vi "Loop (DMA) BAD CHANNELS.vi"(8 "Error IN":errorcluster, 9 "Stop":refnum<vi>, 10 "Sample Rate":u32, 11 "FPGA Ref":T1) -> (0 "Error OUT":errorcluster, 3 "FPGA Ref OUT":T1)   [LabVIEW 2019]
uses:
  <vilib>/rvi/interface/nirviMethod/nirviMethod.xnode
  <vilib>/rvi/errors/niLvFpgaMergeErrorWithErrorCode.vi
  Real-Time/Controls/RT FIFO Mode.ctl
  Type Defs/Pump Data Mode.ctl
  Controls/FPGA_Reference.ctl
  <vilib>/FPGAPlugInAG/Dynamic/niLvFpga_ReadFifo_Dynamic.vi
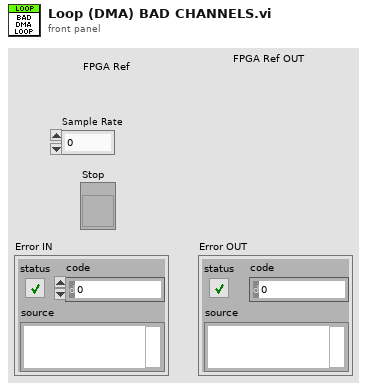
[diagram p1: front panel]
types:
  T1 = typedef "FPGA_Reference.ctl" = refnum<k20>
  T2 = typedef "Pump Data Mode.ctl" = enum16{"Read", "Write Data", "Write Cal", "Write Watlow Data", "Write Pressure Offsets", "Write Initial Times", "Write Pumps Present"}
  T3 = typedef "RT FIFO Mode.ctl" = enum16{"Create", "Write", "Read", "Delete"}
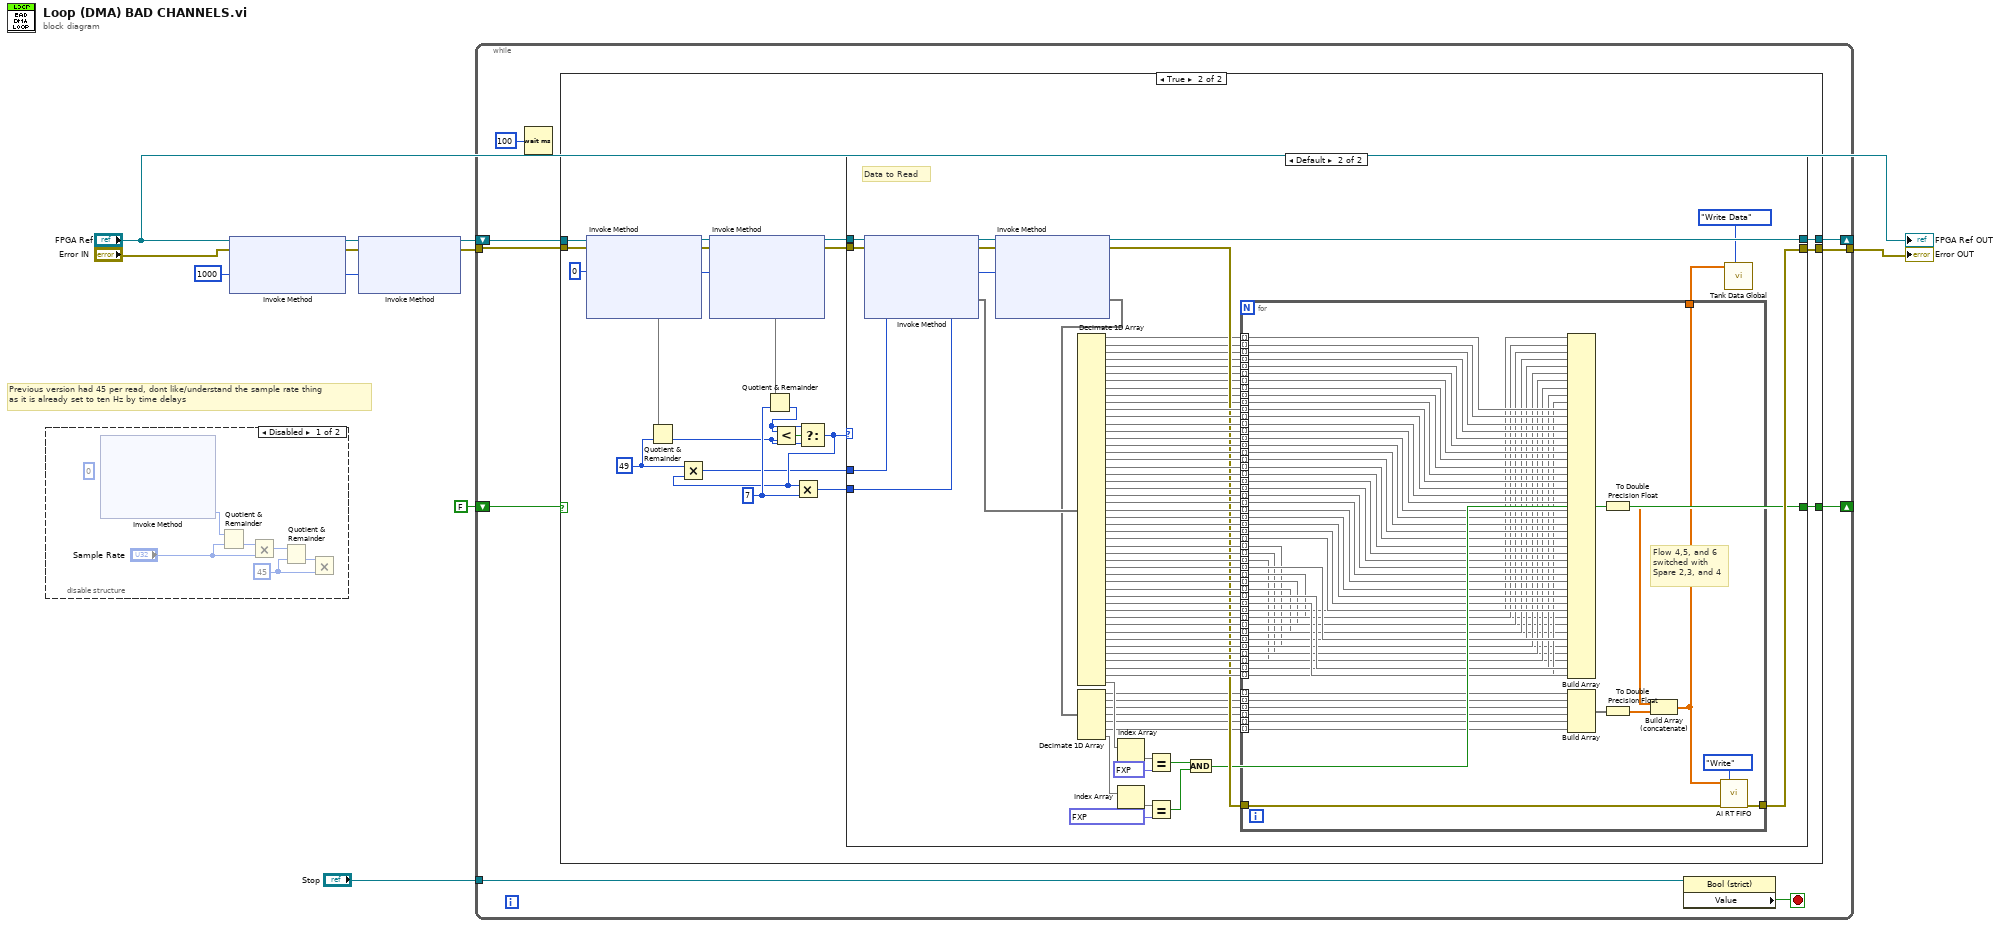
[diagram p0: block diagram]
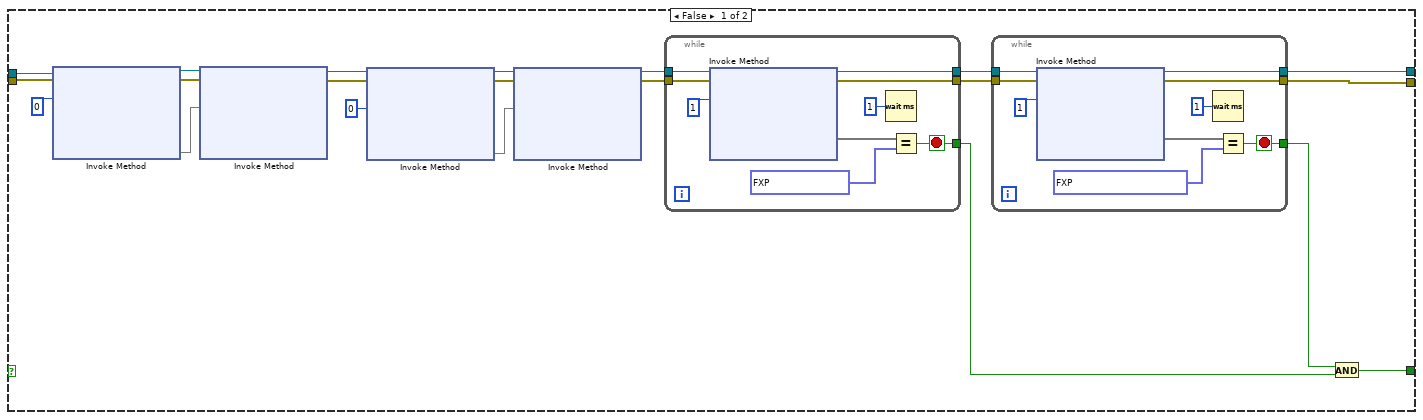
[diagram p3: hidden frame]
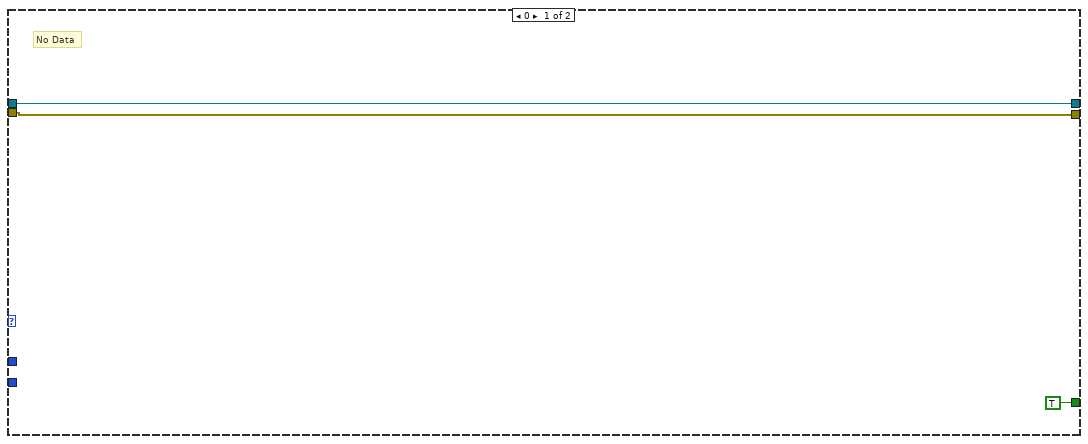
[diagram p4: hidden frame]
diagram:
  w2 = u32 1000 ("Requested Depth")
  # "Previous version had 45 per read, dont like/understand the sample rate thing\nas it is already set to ten Hz by time delays"
  n1 = disable-structure shown="Disabled" {
    frame Disabled {
      w16 = u32 45 ("y")
      w17 = u32 0 ("Number of Elements")
      n2 = xnode "Invoke Method"() -> ("Elements Remaining"=w12:u32)  [unwired: 4 in, 3 out]
      n3 = Quotient & Remainder(x=w12, y="Sample Rate") -> (floor(x/y)=w13:u32)  [unwired: 1 out]
      n4 = Multiply(x=w13, y="Sample Rate") -> (x*y=w14:u32)
      n5 = Quotient & Remainder(x=w14, y=w16) -> (floor(x/y)=w15:u32)  [unwired: 1 out]
      n6 = Multiply(x=w15, y=w16) -> ()  [unwired: 1 out]
    }
    frame Enabled {
    }
  }
  n7 = xnode "Invoke Method"("FPGA VI Reference In"="FPGA Ref", "error in"="Error IN", "Requested Depth"=w2) -> ("FPGA VI Reference Out"=w4:T1, "error out"=w3:errorcluster)  [unwired: 1 out]
  n8 = xnode "Invoke Method"("FPGA VI Reference In"=w4, "error in"=w3, "Requested Depth"=w2) -> ("FPGA VI Reference Out"=w7:T1, "error out"=w6:errorcluster)  [unwired: 1 out]
  n9 = while {
    tunnel: w6 -> [w26]
    tunnel: [w25] -> w9
    shift-right: [w24] -> _
    shift-left: FALSE -> [w23]
    shift-right: [w21] -> _
    shift-left: w7 -> [w22]
    tunnel: "Stop" -> [w20]
    stop <- w19 stop-if-true
    n10 = Wait (ms)(milliseconds to wait=u32 100) -> ()  [unwired: 1 out]
    n11 = case shown="True" w23 {
      tunnel: w26 -> [w47 w85]
      tunnel: [w30 w83] -> w25
      tunnel: [w27 w82] -> w24
      tunnel: w22 -> [w46 w80]
      tunnel: [w31 w81] -> w21
      frame False {
        n12 = xnode "Invoke Method"("FPGA VI Reference In"=w46, "error in"=w47, "Number of Elements"=u32 0) -> ("FPGA VI Reference Out"=w42:T1, "error out"=w44:errorcluster, "Elements Remaining"=w43)  [unwired: 1 in, 1 out]
        n13 = xnode "Invoke Method"("FPGA VI Reference In"=w42, "error in"=w44, "Number of Elements"=w43) -> ("FPGA VI Reference Out"=w39:T1, "error out"=w38:errorcluster)  [unwired: 1 in, 2 out]
        n14 = xnode "Invoke Method"("FPGA VI Reference In"=w39, "error in"=w38, "Number of Elements"=u32 0) -> ("FPGA VI Reference Out"=w37:T1, "error out"=w36:errorcluster, "Elements Remaining"=w41)  [unwired: 1 in, 1 out]
        n15 = xnode "Invoke Method"("FPGA VI Reference In"=w37, "error in"=w36, "Number of Elements"=w41) -> ("FPGA VI Reference Out"=w35:T1, "error out"=w34:errorcluster)  [unwired: 1 in, 2 out]
        n16 = while {
          tunnel: w34 -> [w64]
          tunnel: [w62] -> w32
          tunnel: [w61] -> w28
          tunnel: [w60] -> w33
          tunnel: w35 -> [w59]
          stop <- w61 stop-if-true
          n17 = xnode "Invoke Method"("FPGA VI Reference In"=w59, "error in"=w64, "Number of Elements"=u32 1) -> ("FPGA VI Reference Out"=w60:T1, "error out"=w62:errorcluster, "Data"=w63:void[])  [unwired: 1 in, 1 out]
          n18 = Wait (ms)(milliseconds to wait=u32 1) -> ()  [unwired: 1 out]
          n19 = Equal?(x=w63, y=fxp<+/-,26,15>[] [-9999.0] ("Data")) -> (x = y?=w61:bool)
        }
        n20 = while {
          tunnel: w32 -> [w55]
          tunnel: [w53] -> w30
          tunnel: [w52] -> w29
          tunnel: [w51] -> w31
          tunnel: w33 -> [w50]
          stop <- w52 stop-if-true
          n21 = xnode "Invoke Method"("FPGA VI Reference In"=w50, "error in"=w55, "Number of Elements"=u32 1) -> ("FPGA VI Reference Out"=w51:T1, "error out"=w53:errorcluster, "Data"=w54:void[])  [unwired: 1 in, 1 out]
          n22 = Wait (ms)(milliseconds to wait=u32 1) -> ()  [unwired: 1 out]
          n23 = Equal?(x=w54, y=fxp<+,40,40>[] [1099511627775.0] ("Data")) -> (x = y?=w52:bool)
        }
        n24 = And(x=w29, y=w28) -> (x .and. y?=w27:bool)
      }
      frame True {
        w69 = u32 49 ("y")
        w79 = u32 7 ("y")
        w74 = u32 0 ("Number of Elements")
        n25 = xnode "Invoke Method"("FPGA VI Reference In"=w80, "error in"=w85, "Number of Elements"=w74) -> ("FPGA VI Reference Out"=w78:T1, "error out"=w77:errorcluster, "Elements Remaining"=w84)  [unwired: 1 in, 1 out]
        n26 = Quotient & Remainder(x=w84, y=w69) -> (floor(x/y)=w71:u32)  [unwired: 1 out]
        n27 = xnode "Invoke Method"("FPGA VI Reference In"=w78, "error in"=w77, "Number of Elements"=w74) -> ("FPGA VI Reference Out"=w76:T1, "error out"=w75:errorcluster, "Elements Remaining"=w73)  [unwired: 1 in, 1 out]
        n28 = Quotient & Remainder(x=w73, y=w79) -> (floor(x/y)=w70:u32)  [unwired: 1 out]
        n29 = Less?(x=w70, y=w71) -> (x < y?=w72:bool)
        n30 = Select(t=w70, s=w72, f=w71) -> (s? t:f=w68:u32)
        n31 = Multiply(x=w69, y=w68) -> (x*y=w67:u32)
        n32 = Multiply(x=w68, y=w79) -> (x*y=w66:u32)
        n33 = case shown="Default" w68 {
          tunnel: [w86 w120] -> w81
          tunnel: w75 -> [w88 w164]
          tunnel: [w88 w161] -> w83
          tunnel: [TRUE w100] -> w82
          tunnel: w76 -> [w86 w162]
          tunnel: w67 -> [_ w119]
          tunnel: w66 -> [_ w118]
          frame 0 {
            # "No Data"
          }
          frame Default {
            # "Data to Read"
            n34 = xnode "Invoke Method"("FPGA VI Reference In"=w162, "error in"=w164, "Number of Elements"=w119) -> ("FPGA VI Reference Out"=w121:T1, "error out"=w117:errorcluster, "Data"=w149:void[])  [unwired: 1 in, 1 out]
            n35 = xnode "Invoke Method"("FPGA VI Reference In"=w121, "error in"=w117, "Number of Elements"=w118) -> ("FPGA VI Reference Out"=w120:T1, "error out"=w116:errorcluster, "Data"=w114:void[])  [unwired: 1 in, 1 out]
            n36 = Decimate 1D Array(w149) -> (w89:void[], w90:void[], w91:void[], w92:void[], w93:void[], w94:void[], w95:void[], w96:void[], w97:void[], w98:void[], w160:void[], w159:void[], w158:void[], w157:void[], w156:void[], w155:void[], w154:void[], w153:void[], w152:void[], w151:void[], w150:void[], w148:void[], w147:void[], w146:void[], w145:void[], w144:void[], w143:void[], w142:void[], w141:void[], w140:void[], w139:void[], w138:void[], w137:void[], w136:void[], w135:void[], w134:void[], w133:void[], w132:void[], w131:void[], w130:void[], w129:void[], w128:void[], w127:void[], w126:void[], w125:void[], w124:void[], w123:void[], w122:void[], w115:void[])
            n37 = Decimate 1D Array(w114) -> (w113:void[], w112:void[], w111:void[], w110:void[], w109:void[], w108:void[], w106:void[])
            n38 = Index Array(array=w115) -> (element=w163)  [unwired: 1 in]
            n39 = Index Array(array=w106) -> (element=w105)  [unwired: 1 in]
            n40 = Equal?(x=w163, y=fxp<+/-,26,15> -9999.0) -> (x = y?=w101:bool)
            n41 = Equal?(x=w105, y=fxp<+,40,40> 1099511627775.0) -> (x = y?=w102:bool)
            n42 = And(x=w101, y=w102) -> (x .and. y?=w100:bool)
            n43 = for {
              tunnel: w116 -> [w225]
              tunnel: [w224] -> w161
              tunnel: w160 -> [w220] mode=indexing
              tunnel: w159 -> [w219] mode=indexing
              tunnel: w158 -> [w218] mode=indexing
              tunnel: w157 -> [w223] mode=indexing
              tunnel: w156 -> [w222] mode=indexing
              tunnel: w155 -> [w221] mode=indexing
              tunnel: w154 -> [w217] mode=indexing
              tunnel: w153 -> [w216] mode=indexing
              tunnel: w152 -> [w215] mode=indexing
              tunnel: w151 -> [w202] mode=indexing
              tunnel: w150 -> [w214] mode=indexing
              tunnel: w148 -> [w213] mode=indexing
              tunnel: w147 -> [w212] mode=indexing
              tunnel: w146 -> [w211] mode=indexing
              tunnel: w145 -> [w210] mode=indexing
              tunnel: w144 -> [w209] mode=indexing
              tunnel: w143 -> [w208] mode=indexing
              tunnel: w142 -> [w207] mode=indexing
              tunnel: w141 -> [w206] mode=indexing
              tunnel: w140 -> [w167] mode=indexing
              tunnel: w139 -> [w166] mode=indexing
              tunnel: w138 -> [w165] mode=indexing
              tunnel: [w191] -> w107
              tunnel: w137 -> [w205] mode=indexing
              tunnel: w136 -> [w170] mode=indexing
              tunnel: w135 -> [w169] mode=indexing
              tunnel: w134 -> [w168] mode=indexing
              tunnel: w133 -> [w204] mode=indexing
              tunnel: w132 -> [w203] mode=indexing
              tunnel: w131 -> [w180] mode=indexing
              tunnel: w130 -> [w179] mode=indexing
              tunnel: w129 -> [w178] mode=indexing
              tunnel: w128 -> [w177] mode=indexing
              tunnel: w127 -> [w176] mode=indexing
              tunnel: w126 -> [w175] mode=indexing
              tunnel: w125 -> [w174] mode=indexing
              tunnel: w124 -> [w173] mode=indexing
              tunnel: w123 -> [w172] mode=indexing
              tunnel: w122 -> [w171] mode=indexing
              tunnel: w113 -> [w201] mode=indexing
              tunnel: w112 -> [w200] mode=indexing
              tunnel: w111 -> [w199] mode=indexing
              tunnel: w110 -> [w198] mode=indexing
              tunnel: w109 -> [w197] mode=indexing
              tunnel: w108 -> [w196] mode=indexing
              tunnel: w98 -> [w190] mode=indexing
              tunnel: w97 -> [w189] mode=indexing
              tunnel: w96 -> [w188] mode=indexing
              tunnel: w95 -> [w187] mode=indexing
              tunnel: w94 -> [w186] mode=indexing
              tunnel: w93 -> [w185] mode=indexing
              tunnel: w92 -> [w184] mode=indexing
              tunnel: w91 -> [w183] mode=indexing
              tunnel: w90 -> [w182] mode=indexing
              tunnel: w89 -> [w181] mode=indexing
              # "Flow 4,5, and 6\nswitched with\nSpare 2,3, and 4"
              n44 = Build Array(w180, w179, w178, w177, w176, w175, w174, w173, w172, w171, w181, w182, w183, w184, w185, w186, w187, w188, w189, w190, w220, w219, w218, w223, w222, w221, w217, w216, w215, w202, w214, w213, w212, w211, w210, w209, w208, w207, w206, w170, w169, w168, w205, w167, w166, w165, w204, w203) -> (w195:void[])
              n45 = Build Array(w201, w200, w199, w198, w197, w196) -> (w194:void[])
              n46 = To Double Precision Float(number=w195) -> (double precision float=w193:dbl[])
              n47 = To Double Precision Float(number=w194) -> (double precision float=w192:dbl[])
              n48 = Build Array (concatenate)(w193, w192) -> (w191:dbl[])
              n49 = call "AI RT FIFO.vi"("Data IN"=w191, "Mode"=RT_FIFO_Mode."Write", "Error IN"=w225) -> ("Error OUT"=w224:errorcluster)  [unwired: 10 in, 2 out]
            }
            n50 = call "Tank Data Global.vi"("Pump Data Mode"=Pump_Data_Mode."Write Data", "Tank Data IN"=w107) -> ()  [unwired: 9 in, 1 out]
          }
        }
      }
    }
    n51 = property class="Bool (strict)"(reference=w20) -> ("Value"=w19:bool)  [unwired: 1 in, 2 out]
  }
  "Error OUT" <- w9
  "FPGA Ref OUT" <- "FPGA Ref"
